vi "Receive.vi"(8 "error in (no error)":errorcluster, 10 "Transfer Group in":refnum<class "Transfer Group.lvclass">, 11 "MockTransceiver in":refnum<class "MockTransceiver.lvclass">) -> (0 "error out":errorcluster, 2 "Transfer Group out":refnum<class "Transfer Group.lvclass">, 3 "MockTransceiver out":refnum<class "MockTransceiver.lvclass">)   [LabVIEW 2017, in "MockTransceiver.lvclass"]
uses:
  MockTransceiver.lvclass
  Engine/Classes/Transfer Group/Transfer Group.lvclass
  MockTransceiver.lvclass/MockTransceiver.ctl
  Engine/Classes/Transceiver/Transceiver.lvclass
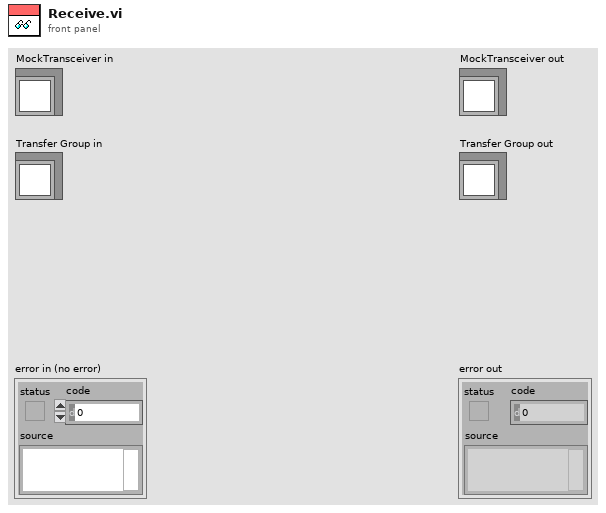
[diagram p1: front panel]
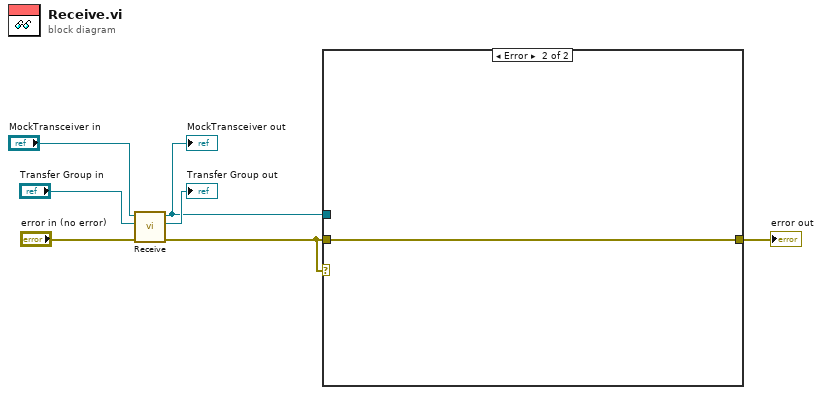
[diagram p0: block diagram]
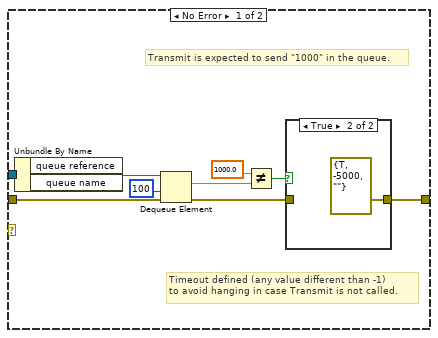
[diagram p2: hidden frame]
diagram:
  n1 = call-parent "Receive.vi"("error in (no error)"="error in (no error)", "Transfer Group in"="Transfer Group in", "Transceiver in"="MockTransceiver in") -> ("error out"=w1:errorcluster, "Transfer Group out"=→"Transfer Group out":refnum<class "Transfer Group.lvclass">, "Transceiver out"=w2:refnum<class "MockTransceiver.lvclass">)  [unwired: 6 in]
  "MockTransceiver out" <- w2
  n2 = case shown="Error" w1 {
    tunnel: [w10 w19] -> w3
    tunnel: w1 -> [w9 w19]
    tunnel: w2 -> [w8 _]
    frame No Error {
      # "Transmit is expected to send \"1000\" in the queue."
      # "Timeout defined (any value different than -1)\nto avoid hanging in case Transmit is not called."
      n3 = Unbundle By Name(w8) -> ("queue reference"=w16:refnum<queue>)  [unwired: 1 out]
      n4 = Dequeue Element(queue=w16, timeout in ms (-1)=100, error in (no error)=w9) -> (element=w15:dbl, error out=w12:errorcluster)  [unwired: 2 out]
      n5 = Not Equal?(x=1000.0, y=w15) -> (x != y?=w13:bool)
      n6 = case shown="True" w13 {
        tunnel: [w17 errorcluster {"status"=TRUE, "code"=-5000, "source"=""} ("error constant")] -> w10
        tunnel: w12 -> [w17 _]
        frame False {
        }
        frame True {
        }
      }
    }
    frame Error {
    }
  }
  "error out" <- w3
